vi "fix_shared_library_paths_for_folder.vi"(8 "error in":errorcluster, 11 "Folder of VIs":path=path "C:/Projects/reqwest-rs-labview/jki_lib_reqwest_rs_labview-0.1.0.1/File Group 0/vi.lib/JKI/reqwest-rs-labview") -> (0 "error out":errorcluster)   [LabVIEW 2020]
uses:
  <vilib>/Utility/traverseref.llb/TRef TravTarget.ctl
  <vilib>/Utility/traverseref.llb/VI Scripting - Traverse.lvlib
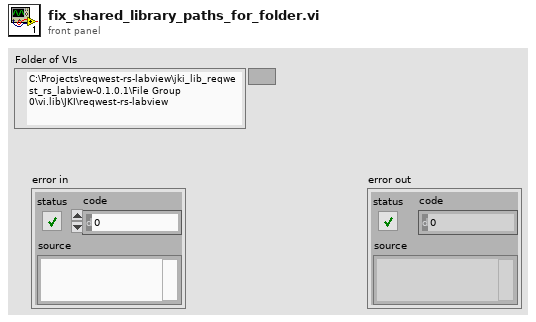
[diagram p1: front panel]
types:
  T1 = typedef "TRef TravTarget.ctl" = enum16{"FP", "BD", "Other"}
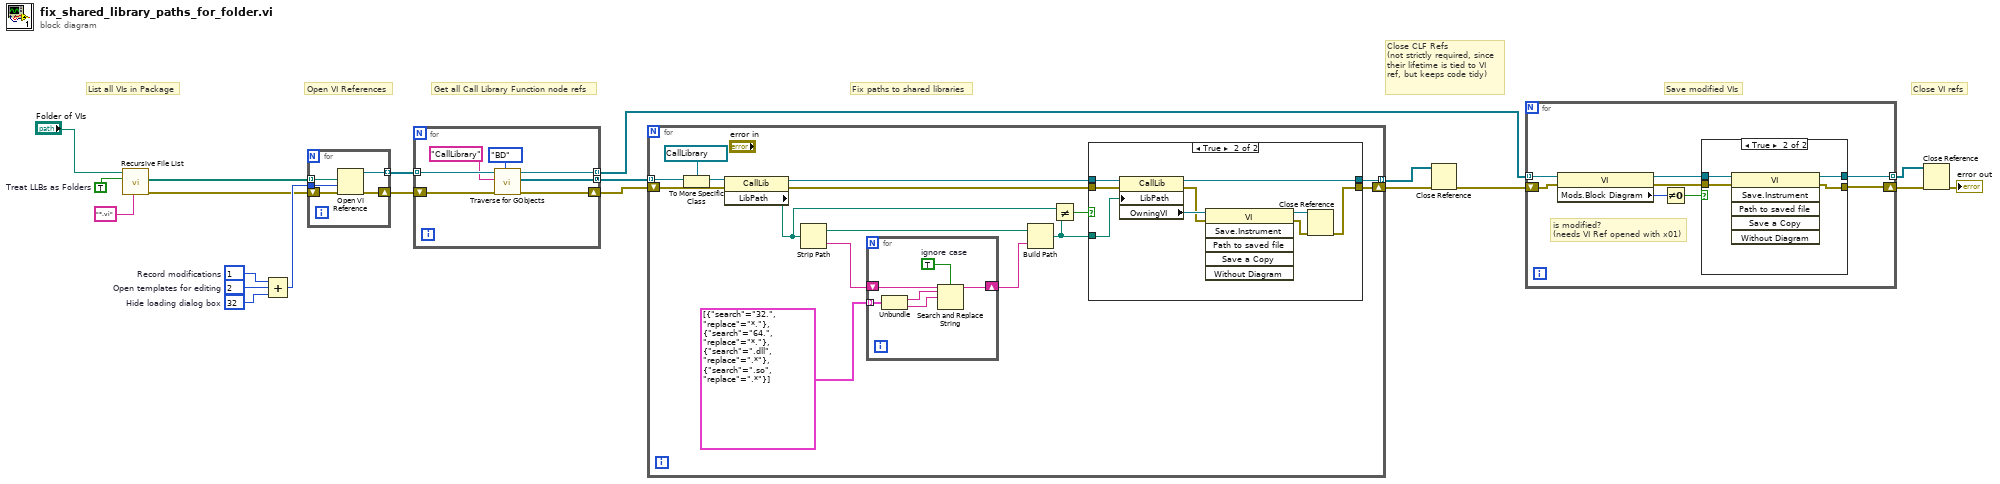
[diagram p0: block diagram]
diagram:
  w11 = 32  # Hide loading dialog box
  w13 = 2  # Open templates for editing
  w12 = 1  # Record modifications
  w19 = TRUE  # Treat LLBs as Folders
  # "Close CLF Refs\n(not strictly required, since their lifetime is tied to VI ref, but keeps code tidy)"
  # "Close VI refs"
  # "List all VIs in Package"
  # "Open VI References"
  # "Save modified VIs"
  # "Fix paths to shared libraries"
  # "Get all Call Library Function node refs"
  n1 = call <vilib>:"Recursive File List.vi"("pattern"="*.vi", "Treat LLBs as Folders?"=w19, "Folder Path"="Folder of VIs") -> ("error out"=w7:errorcluster, "All Files in Dir"=w17:path[])  [unwired: 4 in, 3 out]
  n2 = Compound Arithmetic op=unknown(w12, w13, w11) -> (w10:i32)
  n3 = for {
    tunnel: w17 -> [w25] mode=indexing
    tunnel: [w24] -> w16 mode=indexing
    tunnel: w10 -> [w23]
    shift-right: [w22] -> w8
    shift-left: w7 -> [w21]
    n4 = Open VI Reference(vi path=w25, options=w23, error in (no error)=w21) -> (vi reference=w24:refnum<vi>, error out=w22:errorcluster)  [unwired: 3 in]
  }
  n5 = for {
    tunnel: w16 -> [w32] mode=indexing
    tunnel: [w30] -> w15 mode=concatenating
    tunnel: [w28] -> w14 mode=indexing
    shift-right: [w27] -> w9
    shift-left: w8 -> [w26]
    n6 = call <vilib>:"Traverse for GObjects.vi"("Traverse Target"=TRef_TravTarget."BD", "error in (no error)"=w26, "Class Name"="CallLibrary", "VI Refnum"=w32) -> ("error out"=w27:errorcluster, "References"=w30:refnum<vi>[], "dup VI Refnum"=w28:refnum<vi>)  [unwired: 4 in, 1 out]
  }
  n7 = for {
    tunnel: w15 -> [w47] mode=indexing
    shift-right: [w39] -> w5
    shift-left: w9 -> [w37]
    tunnel: [w36] -> w6 mode=indexing
    n8 = To More Specific Class(target class=refnum<vi> refnum ("Other Refnum"), reference=w47) -> (specific class reference=w45:refnum<vi>)  [unwired: 1 in, 1 out]
    n9 = property class="CallLib"(reference=w45, error in=w37) -> (reference out=w40:refnum<vi>, error out=w38:errorcluster, "LibPath"=w34:path)
    n10 = Strip Path(path=w34) -> (stripped path=w41:path, name=w44:string)
    n11 = for {
      tunnel: cluster{"search":string, "replace":string}[] [{"search"="32.", "replace"="*."}, {"search"="64.", "replace"="*."}, {"search"=".dll", "replace"=".*"}, {"search"=".so", "replace"=".*"}] -> [w63] mode=indexing
      shift-right: [w59] -> w42
      shift-left: w44 -> [w64]
      w60 = TRUE  # ignore case
      n12 = Unbundle(w63) -> ("search"=w62:string, "replace"=w61:string)
      n13 = Search and Replace String(case sensitive?=w60, input string=w64, search string=w62, replace string=w61) -> (result string=w59:string)  [unwired: 4 in, 3 out]
    }
    n14 = Build Path(base path=w41, name or relative path=w42) -> (appended path=w35:path)
    n15 = Not Equal?(x=w34, y=w35) -> (x != y?=w33:bool)
    n16 = case shown="True" w33 {
      tunnel: w40 -> [w49 w58]
      tunnel: [w48 w51] -> w39
      tunnel: w38 -> [w48 w57]
      tunnel: [w49 w50] -> w36
      tunnel: w35 -> [_ w56]
      frame False {
      }
      frame True {
        n17 = property class="CallLib"(reference=w58, error in=w57, "LibPath"=w56) -> (reference out=w50:refnum<vi>, error out=w52:errorcluster, "OwningVI"=w55:refnum<vi>)
        n18 = invoke class="VI" method="Save.Instrument"(reference=w55, error in=w52) -> (reference out=w53:refnum<vi>, error out=w54:errorcluster)  [unwired: 4 in, 4 out]
        n19 = Close Reference(reference=w53, error in (no error)=w54) -> (error out=w51:errorcluster)
      }
    }
  }
  n20 = Close Reference(reference=w6, error in (no error)=w5) -> (error out=w4:errorcluster)
  n21 = for {
    tunnel: w14 -> [w72] mode=indexing
    tunnel: [w69] -> w2 mode=indexing
    shift-right: [w66] -> w3
    shift-left: w4 -> [w67]
    # "is modified?\n(needs VI Ref opened with x01)"
    n22 = property class="VI"(reference=w72, error in=w67) -> (reference out=w70:refnum<vi>, error out=w65:errorcluster, "Mods.Block Diagram"=w71:u32)
    n23 = Not Equal To 0?(x=w71) -> (x != 0?=w68:bool)
    n24 = case shown="True" w68 {
      tunnel: w70 -> [w74 w78]
      tunnel: [w74 w77] -> w69
      tunnel: [w73 w75] -> w66
      tunnel: w65 -> [w73 w76]
      frame False {
      }
      frame True {
        n25 = invoke class="VI" method="Save.Instrument"(reference=w78, error in=w76) -> (reference out=w77:refnum<vi>, error out=w75:errorcluster)  [unwired: 4 in, 4 out]
      }
    }
  }
  n26 = Close Reference(reference=w2, error in (no error)=w3) -> (error out=→"error out":errorcluster)
